vi "simple_subscriber.vi"() -> ()   [LabVIEW 2014]
panel:
  out "JSON字符串 2":string
  in  "停止":bool
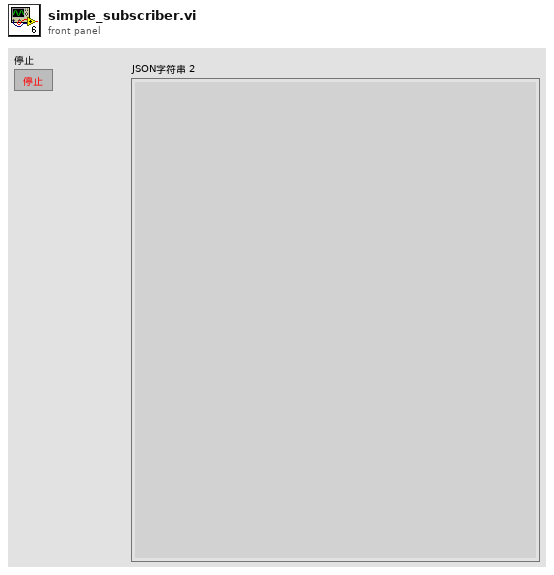
[diagram p1: front panel]
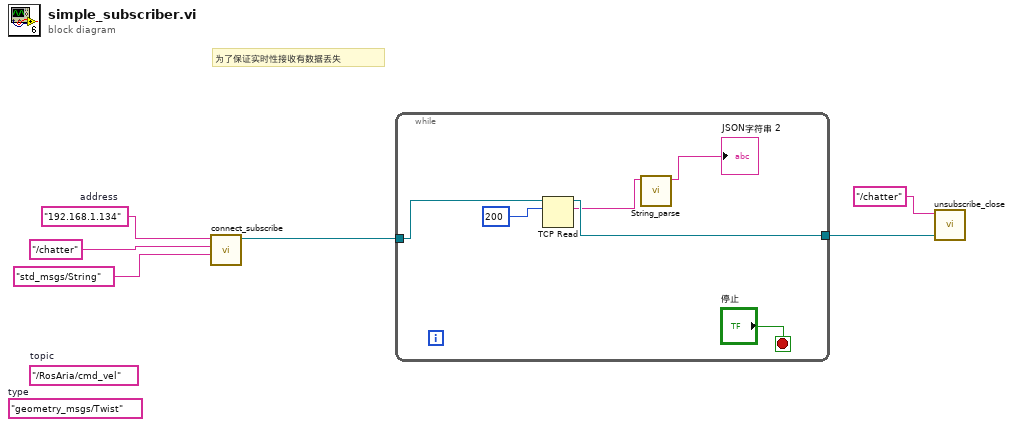
[diagram p0: block diagram]
diagram:
  (unwired) "geometry_msgs/Twist"  # type
  (unwired) "/RosAria/cmd_vel"  # topic
  w6 = "192.168.1.134"  # address
  # "为了保证实时性接收有数据丢失"
  n1 = call "connect_subscribe.vi"("type"="std_msgs/String", "topic"="/chatter", "address"=w6) -> ("连接ID输出"=w5:refnum<k5>)  [unwired: 7 in, 1 out]
  n2 = while {
    tunnel: [w12] -> w2
    tunnel: w5 -> [w9]
    stop <- "停止" stop-if-true
    n3 = TCP Read(connection ID=w9, bytes to read=200 ("读取的字节")) -> (connection ID out=w12:refnum<k5>, data out=w7:string)  [unwired: 3 in, 1 out]
    n4 = call "String_parse.vi"("字符串"=w7) -> ("data"=→"JSON字符串 2":string)  [unwired: 9 in, 1 out]
  }
  n5 = call "unsubscribe_close.vi"("连接ID"=w2, "topic"="/chatter") -> ()  [unwired: 10 in]
